vi "ActualizarTablaNivelPresionSonora.vi"(8 "error in (no error)":errorcluster, 10 "medido":dbl, 11 "Prueba21_1":refnum<class "Prueba21.lvclass">) -> (0 "error out":errorcluster, 3 "Prueba21_1":refnum<class "Prueba21.lvclass">)   [LabVIEW 2019, in "Prueba21.lvclass"]
uses:
  Prueba21.lvclass
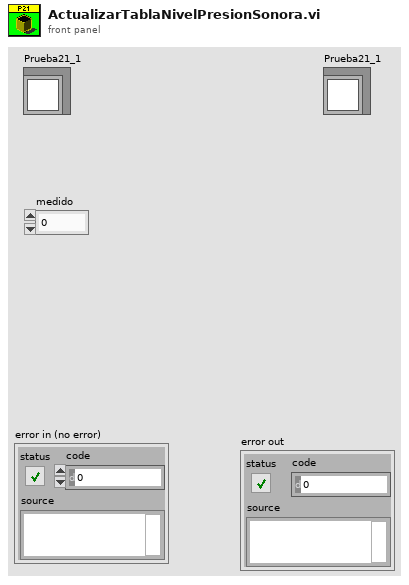
[diagram p1: front panel]
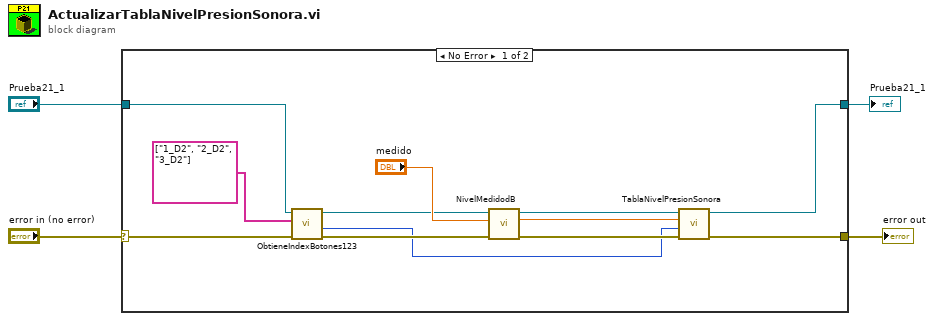
[diagram p0: block diagram]
diagram:
  n1 = case shown="No Error" "error in (no error)" {
    selector: "error in (no error)" -> [w10 w17]
    tunnel: [w16 w18] -> w4
    tunnel: [w11 w17] -> w3
    tunnel: "Prueba21_1" -> [w7 w18]
    frame No Error {
      n2 = call "ObtieneIndexBotones123.vi"("error in (no error)"=w10, "Botones"=string[] ["1_D2", "2_D2", "3_D2"] ("String"), "Prueba21_1 in"=w7) -> ("error out"=w9:errorcluster, "index of element"=w5:i32, "Prueba21_1 out"=w8:refnum<class "Prueba21.lvclass">)  [unwired: 6 in]
      n3 = call "NivelMedidodB.vi"("error in (no error)"=w9, "Voltaje"="medido", "Prueba21 in"=w8) -> ("error out"=w13:errorcluster, "Nivel Medido [dB]"=w14:dbl, "Prueba21 out"=w15:refnum<class "Prueba21.lvclass">)  [unwired: 6 in]
      n4 = call "TablaNivelPresionSonora.vi"("error in (no error)"=w13, "fila"=w5, "NivelMedido"=w14, "Prueba21_1 in"=w15) -> ("error out"=w11:errorcluster, "Prueba21_1 out"=w16:refnum<class "Prueba21.lvclass">)  [unwired: 6 in]
    }
    frame Error {
    }
  }
  "Prueba21_1" <- w4
  "error out" <- w3
